vi "SPARK Open.vi"   [LabVIEW 2023]
doc: "Open the SPARK motor controller.\n\n<b>Device Number</b> is the CAN ID of the controller. Use a value between 1 and 62.\n\n<b>Invert</b> will tell the LabVIEW driver to invert the output of the motor. For a device that is configured as a Follower, this flag will configure the follower to driver opposite of the Leader controller."
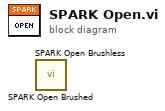
[diagram p0: block diagram]
diagram:
  n1 = call "SPARK Open Brushed.vi"() -> ()  [unwired: 10 in, 2 out]
  n2 = call "SPARK Open Brushless.vi"() -> ()  [unwired: 10 in, 2 out]
